vi "svfa_Build Spectrum Info (N Ch).vi"(0 "scaled signal(s)":waveform(dbl)[](array[waveform]), 1 "processing control in":T8(ring), 5 "window":T7 items=["None"=0, "Hanning"=1, "Hamming"=2, "Blackman-Harris"=3, "Exact Blackman"=4, "Blackman"=5, "Flat Top"=6, "4 Term B-Harris "=7, "7 Term B-Harris"=8, "Low Sidelobe"=9, "Force"=64, "Exponential"=65, "Blackman Nuttall"=11, "Triangle"=30, "Bartlett-Hanning"=31, "Bohman"=32, "Parzen"=33, "Welch"=34, "Kaiser"=60, "Dolph-Chebyshev"=61, "Gaussian"=62], 7 "window size":i32, 9 "spectra info in":T1[](array[typedef]) {"x-axis units" items=["Time (s)"=0, "Frequency-CB (Hz)"=1, "Frequency-CPB (Hz)"=1248, "Frequency-Arbitrary (Hz)"=2357, "Quefrency (s)"=2, "Revolutions (rev)"=3, "Order"=4, "Speed (RPM)"=11, "Speed (rad/s)"=21, "Index"=65535]; "weighting filter" items=["Linear", "A-weighting", "B-weighting", "C-weighting", "ITU-R 468-4", "Dolby", "CCITT", "C-message", "Wb", "Wc", "Wd", "We", "Wf", "Wh", "Wj", "Wk", "Wm", "AES17 20 kHz lowpass", "AES17 40 kHz lowpass", "AES17 20 kHz highpass", "AES17 40 kHz highpass"]; "dB reference [EU]" format="%.2f"; "engineering units" items=["custom..."=0, "V"=1, "A"=21, "C"=30, "pC"=31, "s"=32, "-"=29, "Pa"=2, "N"=20, "g"=3, "m/s^2"=4, "m/s"=5, "m"=6, "mm/s"=12, "mm"=13, "micron/s"=14, "micron"=15, "in/s^2"=7, "in/s"=8, "in"=9, "mil/s"=10, "mil"=11, "rad/s^2"=16, "rad/s"=17, "rad"=18, "deg/s^2"=26, "deg/s"=27, "deg"=28, "RPM"=22, "cycle/s^2"=23, "Hz"=24, "cycle"=25, "strain"=19]; "spectral info"."window" items=["None "=0, "Hanning"=1, "Hamming"=2, "Blackman-Harris"=3, "Exact Blackman"=4, "Blackman"=5, "Flat Top"=6, "4 Term B-Harris "=7, "7 Term B-Harris"=8, "Low Sidelobe"=9, "Force - Exponential"=10, "Gaussian"=62]}, 11 "error in (no error)":errorcluster, 12 "spectrum type":T3=enum."Power [Magnitude^2]", 13 "x-axis units":u16(ring)=1 items=["time"=0, "frequency"=1, "quefrency"=2, "revolutions"=3, "order"=4, "rpm"=11], 14 "spectral density?":bool) -> (3 "dup processing control":T8(ring), 4 "dup scaled signals":waveform(dbl)[](array[waveform]), 10 "spectra info out":T1[](array[typedef]) {"x-axis units" items=["Time (s)"=0, "Frequency-CB (Hz)"=1, "Frequency-CPB (Hz)"=1248, "Frequency-Arbitrary (Hz)"=2357, "Quefrency (s)"=2, "Revolutions (rev)"=3, "Order"=4, "Speed (RPM)"=11, "Speed (rad/s)"=21, "Index"=65535]; "weighting filter" items=["Linear", "A-weighting", "B-weighting", "C-weighting", "ITU-R 468-4", "Dolby", "CCITT", "C-message", "Wb", "Wc", "Wd", "We", "Wf", "Wh", "Wj", "Wk", "Wm", "AES17 20 kHz lowpass", "AES17 40 kHz lowpass", "AES17 20 kHz highpass", "AES17 40 kHz highpass"]; "dB reference [EU]" format="%.2f"; "engineering units" items=["custom..."=0, "V"=1, "A"=21, "C"=30, "pC"=31, "s"=32, "-"=29, "Pa"=2, "N"=20, "g"=3, "m/s^2"=4, "m/s"=5, "m"=6, "mm/s"=12, "mm"=13, "micron/s"=14, "micron"=15, "in/s^2"=7, "in/s"=8, "in"=9, "mil/s"=10, "mil"=11, "rad/s^2"=16, "rad/s"=17, "rad"=18, "deg/s^2"=26, "deg/s"=27, "deg"=28, "RPM"=22, "cycle/s^2"=23, "Hz"=24, "cycle"=25, "strain"=19]; "spectral info"."window" items=["None "=0, "Hanning"=1, "Hamming"=2, "Blackman-Harris"=3, "Exact Blackman"=4, "Blackman"=5, "Flat Top"=6, "4 Term B-Harris "=7, "7 Term B-Harris"=8, "Low Sidelobe"=9, "Force - Exponential"=10, "Gaussian"=62]}, 15 "error out":errorcluster)   [LabVIEW 2017]
uses:
  <vilib>/addons/_NISVFA/_Shared subVIs/Controls/svc_Window.ctl
  <vilib>/addons/_NISVFA/_Shared subVIs/Controls/svc_Spectrum Type.ctl
  <vilib>/addons/_NISVFA/_Shared subVIs/Controls/svc_Spectrum Info.ctl
  <vilib>/addons/_NISVFA/_Shared subVIs/Controls/svc_X-Axis Units.ctl
  <vilib>/addons/_NISVFA/_Shared subVIs/Controls/svc_Engineering Units Text Ring.ctl
  <vilib>/addons/_NISVFA/_Shared subVIs/Controls/svc_Weighting Filter Text Ring.ctl
  <vilib>/addons/_NISVFA/_Shared subVIs/Controls/svc_Complimentary Spectrum Units.ctl
  <vilib>/addons/_NISVFA/_Shared subVIs/Common/svc_Get SV Channel Info.vi
  <vilib>/addons/_NISVFA/_Shared subVIs/Common/svc_Spectrum Units.vi
  <vilib>/addons/_NISVFA/_Shared subVIs/Common/svc_Get Weighting Enum and Labels.vi
  <vilib>/addons/_NISVFA/_Shared subVIs/Common/svc_Unit Label Lexical Class.vi
  <vilib>/addons/_NISVFA/_Shared subVIs/Common/svc_Engineering Units to Unit Label.vi
  <vilib>/addons/_NISVFA/_Shared subVIs/Common/svc_Format Value (DBL).vi
  <vilib>/addons/_NISVFA/_Shared subVIs/Common/svc_Channel Info to Spectrum Info.vi
  <vilib>/addons/_NISVFA/_Shared subVIs/Common/svc_Unit Label to Engineering Units.vi
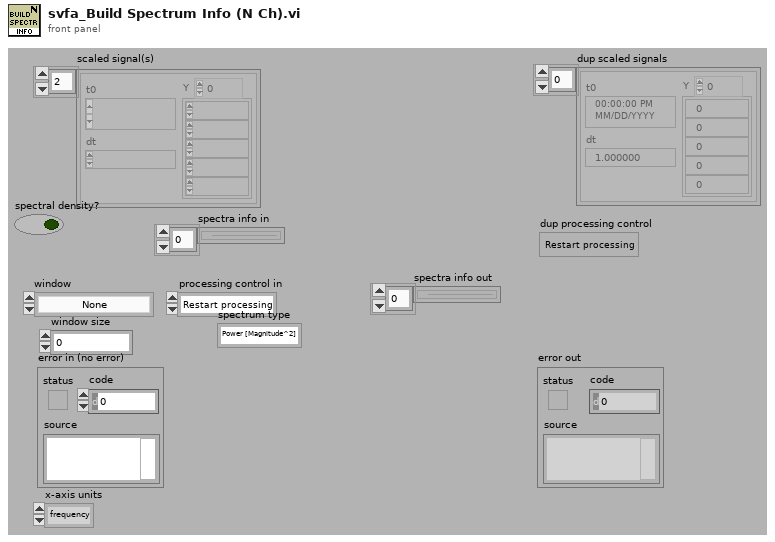
[diagram p1: front panel]
types:
  T1 = typedef "svc_Spectrum Info.ctl" = cluster{"channel name":string, "description":string, "x-axis units":T2, "spectral info":cluster{"spectrum type":T3, "linear/dB":enum16{"linear", "dB"}, "window":u16, "window size":i32, "FFT size":i32}, "engineering units":T4, "custom label":string, "dB reference [EU]":dbl, "peak units":enum16{"rms", "peak", "peak-peak"}, "weighting filter":T5, "spectral density?":bool, "unit label":string, "spectrum skewed?":bool, "complimentary spectrum units":T6}
  T2 = typedef "svc_X-Axis Units.ctl" = u16
  T3 = typedef "svc_Spectrum Type.ctl" = enum16{"FFT Spectrum [complex]", "Amplitude [Magnitude]", "Power [Magnitude^2]", "Cross Spectrum [complex]", "Frequency Response [Complex]"}
  T4 = typedef "svc_Engineering Units Text Ring.ctl" = u16
  T5 = typedef "svc_Weighting Filter Text Ring.ctl" = u16
  T6 = typedef "svc_Complimentary Spectrum Units.ctl" = enum16{"none", "radians", "degrees", "cycles", "imaginary"}
  T7 = typedef "svc_Window.ctl" = u32
  T8 = enum16{"Restart processing", "Continue processing", "Skip processing"}
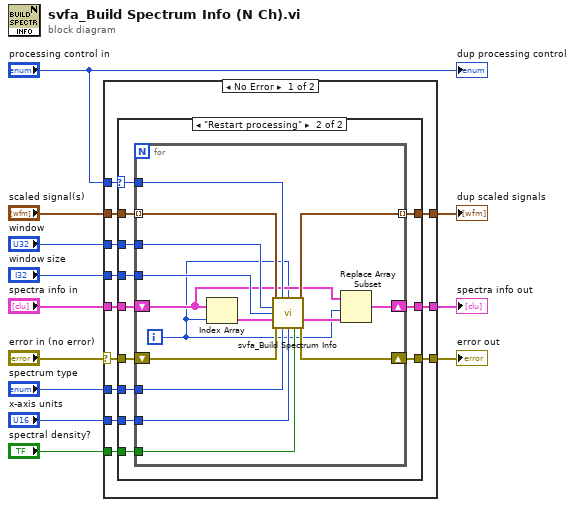
[diagram p0: block diagram]
diagram:
  n1 = case shown="No Error" "error in (no error)" {
    selector: "error in (no error)" -> [w18 w57]
    tunnel: "window" -> [w24 _]
    tunnel: "window size" -> [w23 _]
    tunnel: "spectrum type" -> [w22 _]
    tunnel: "scaled signal(s)" -> [w21 w56]
    tunnel: "processing control in" -> [w13 _]
    tunnel: [w20 w57] -> w7
    tunnel: [w19 w55] -> w6
    tunnel: [w17 w56] -> w4
    tunnel: "x-axis units" -> [w16 _]
    tunnel: "spectra info in" -> [w15 w55]
    tunnel: "spectral density?" -> [w14 _]
    frame No Error {
      n2 = case shown="\"Restart processing\"" w13 {
        selector: w13 -> [_ w28]
        tunnel: w24 -> [_ w39]
        tunnel: w23 -> [_ w38]
        tunnel: w22 -> [_ w37]
        tunnel: w21 -> [w27 w36]
        tunnel: [w25 w35] -> w20
        tunnel: [w26 w34] -> w19
        tunnel: w18 -> [w25 w33]
        tunnel: [w27 w32] -> w17
        tunnel: w16 -> [_ w31]
        tunnel: w15 -> [w26 w30]
        tunnel: w14 -> [_ w29]
        frame Default {
        }
        frame "Restart processing" {
          n3 = for {
            tunnel: w36 -> [w45] mode=indexing
            tunnel: w37 -> [w47]
            tunnel: w39 -> [w49]
            tunnel: w38 -> [w48]
            shift-right: [w50] -> w35
            shift-left: w33 -> [w51]
            tunnel: [w44] -> w32 mode=indexing
            tunnel: w31 -> [w46]
            tunnel: w28 -> [w54]
            shift-right: [w42] -> w34
            shift-left: w30 -> [w43]
            tunnel: w29 -> [w41]
            i -> [w40]
            n4 = Index Array(array=w43, index=w40) -> (element=w53:T1)
            n5 = call <vilib>:"svfa_Build Spectrum Info.vi"("scaled signal [EU]"=w45, "processing control"=w54, "channel index"=w40, "window"=w49, "window size"=w48, "spectrum info in"=w53, "error in (no error)"=w51, "spectrum type"=w47, "x-axis units"=w46, "spectral density?"=w41) -> ("dup scaled signal [EU]"=w44:waveform(dbl), "spectrum info out"=w52:T1, "error out"=w50:errorcluster)  [unwired: 2 in, 1 out]
            n6 = Replace Array Subset(array=w43, new element=w52, index=w40) -> (w42:T1[])
          }
        }
      }
    }
    frame Error {
    }
  }
  "error out" <- w7
  "spectra info out" <- w6
  "dup scaled signals" <- w4
  "dup processing control" <- "processing control in"
